vi "CheckServerRunningStatus.vi"(3 "ROS":T1) -> (1 "running?":bool)   [LabVIEW 2012]
uses:
  <userlib>/ROSforLV/ROS/Code/SubVIs/_ROSControl.ctl
  <userlib>/ROSforLV/ROS/Code/SubVIs/_ROSDirection.ctl
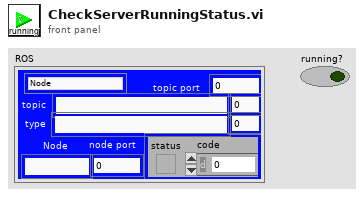
[diagram p1: front panel]
types:
  T1 = typedef "_ROSControl.ctl" = cluster{"topic port":u16, "Node":string, "topic":string, "type":string, "node port":u16, "error ":errorcluster, "Direction":T2, "Update (ms)":u16, "queue size":u16}
  T2 = typedef "_ROSDirection.ctl" = enum16{"Node", "Publisher", "Subscriber", "Service Client"}
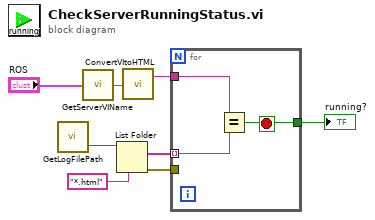
[diagram p0: block diagram]
diagram:
  n1 = call <userlib>:"GetLogFilePath.vi"() -> ("LogFolder"=w5:path)  [unwired: 2 in, 1 out]
  n2 = call <userlib>:"GetServerVIName.vi"("ROS"="ROS") -> ("vi name"=w2:string)
  n3 = List Folder(path=w5, pattern="*.html") -> (filenames=w7:string[], error out=w8:errorcluster)  [unwired: 2 in, 2 out]
  n4 = call <userlib>:"ConvertVItoHTML.vi"("vi name"=w2) -> ("Htm log name"=w3:string)  [unwired: 1 out]
  n5 = for {
    tunnel: w3 -> [w11]
    tunnel: [w10] -> w4
    tunnel: w7 -> [w9] mode=indexing
    tunnel: w8 -> [_]
    stop <- w10 stop-if-true
    n6 = Equal?(x=w11, y=w9) -> (x = y?=w10:bool)
  }
  "running?" <- w4
